vi "Pos_def.vi"() -> ()   [LabVIEW 2017]
panel:
  in  "Pos_def":T1
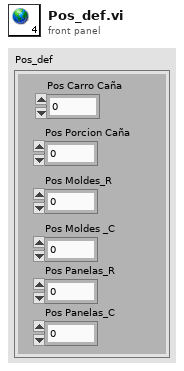
[diagram p1: front panel]
types:
  T1 = cluster{"Pos Carro Caña":i32, "Pos Porcion Caña ":i32, "Pos Moldes_R":i32, "Pos Panelas_R":i32, "Pos Panelas_C":i32, "Pos Moldes _C":i32}
diagram:
